vi "SwerveMain.vi"   [LabVIEW 2017]
uses:
  <vilib>/Rock Robotics/Network Tables/NT Read Boolean.vi
  SwerveGlobals.vi
types:
  T1 = typedef "WPI_MotorControlDeviceRef.ctl" = cluster{"DeviceStatus":errorcluster, "Type":T2, "PWM":cluster{"PWM Channel":T3, "DeadBand":T4}, "CAN":cluster{"Device Number":u8, "SetOutput VI Ref":variant, "GetOutput VI Ref":variant, "Enable VI Ref":variant, "Disable VI Ref":variant, "Data":variant}, "Invert":bool, "DIO PWM":cluster{"PWM \"Enable\" Channel":T3, "DIOChannel":T5, "PWM Rate":dbl}}
  T2 = typedef "WPI_MotorControlType.ctl" = enum16{"PWM", "CAN", "DIO PWM"}
  T3 = typedef "FPGA_DIOPWMChannel.ctl" = enum8{"PWM 0", "PWM 1", "PWM 2", "PWM 3", "PWM 4", "PWM 5", "PWM 6", "PWM 7", "PWM 8", "PWM 9", "PWM MXP 0", "PWM MXP 1", "PWM MXP 2", "PWM MXP 3", "PWM MXP 4", "PWM MXP 5", "PWM MXP 6", "PWM MXP 7", "PWM MXP 8", "PWM MXP 9", "Invalid"}
  T4 = typedef "WPI_PWMDeadband.ctl" = cluster{"Name":string, "maxPositivePwm":i32, "minPositivePwm":i32, "centerPwm":i32, "maxNegativePwm":i32, "minNegativePwm":i32, "angularRange":u16}
  T5 = typedef "FPGA_DIOChannel.ctl" = enum8{"DIO 0", "DIO 1", "DIO 2", "DIO 3", "DIO 4", "DIO 5", "DIO 6", "DIO 7", "DIO 8", "DIO 9", "DIO MXP 0", "DIO MXP 1", "DIO MXP 2", "DIO MXP 3", "DIO MXP 4", "DIO MXP 5", "DIO MXP 6", "DIO MXP 7", "DIO MXP 8", "DIO MXP 9", "DIO MXP 10", "DIO MXP 11", "DIO MXP 12", "DIO MXP 13", "DIO MXP 14", "DIO MXP 15", "SPI Port CS1", "SPI Port CS2", "SPI Port CS3", "SPI Port MISO", "SPI Port MOSI", "Invalid"}
  T6 = typedef "WPI_AnalogChannelDevRef.ctl" = cluster{"DevStatus":errorcluster, "Analog Channel":T7}
  T7 = typedef "FPGA_AIChannel.ctl" = enum8{"AI 0", "AI 1", "AI 2", "AI 3", "AI MXP 0", "AI MXP 1", "AI MXP 2", "AI MXP 3", "Invalid"}
  T8 = cluster{"MotorControlDevRef":T1, "MotorControlDevRef":T1, "MotorControlDevRef":T1, "MotorControlDevRef":T1}
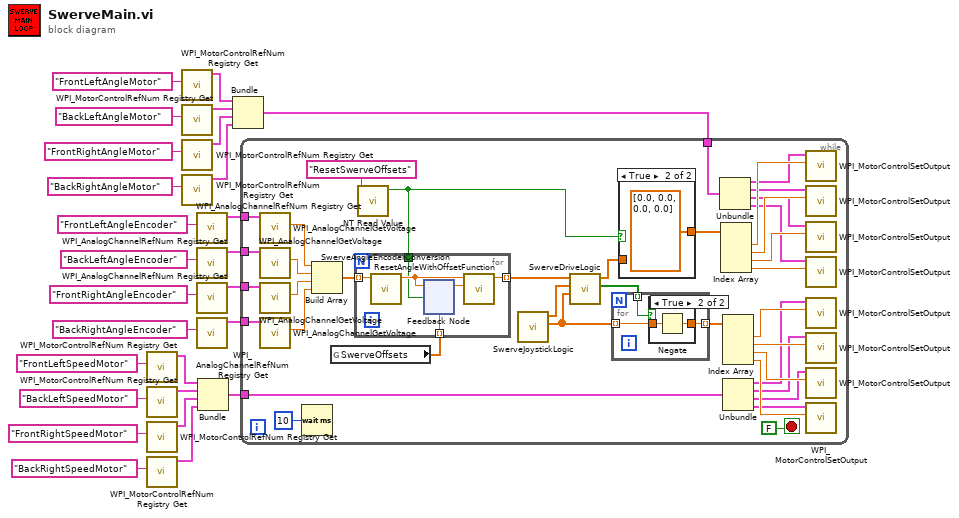
[diagram p0: block diagram]
diagram:
  n1 = call <vilib>:"WPI_MotorControlRefNum Registry Get.vi"("refnum name"="FrontLeftSpeedMotor") -> ("MotorControlDevRef"=w4:T1)  [unwired: 9 in, 1 out]
  n2 = call <vilib>:"WPI_MotorControlRefNum Registry Get.vi"("refnum name"="BackLeftSpeedMotor") -> ("MotorControlDevRef"=w12:T1)  [unwired: 9 in, 1 out]
  n3 = call <vilib>:"WPI_MotorControlRefNum Registry Get.vi"("refnum name"="FrontRightSpeedMotor") -> ("MotorControlDevRef"=w13:T1)  [unwired: 9 in, 1 out]
  n4 = call <vilib>:"WPI_MotorControlRefNum Registry Get.vi"("refnum name"="BackRightSpeedMotor") -> ("MotorControlDevRef"=w14:T1)  [unwired: 9 in, 1 out]
  n5 = call <vilib>:"WPI_MotorControlRefNum Registry Get.vi"("refnum name"="FrontLeftAngleMotor") -> ("MotorControlDevRef"=w1:T1)  [unwired: 9 in, 1 out]
  n6 = call <vilib>:"WPI_MotorControlRefNum Registry Get.vi"("refnum name"="BackLeftAngleMotor") -> ("MotorControlDevRef"=w5:T1)  [unwired: 9 in, 1 out]
  n7 = call <vilib>:"WPI_MotorControlRefNum Registry Get.vi"("refnum name"="FrontRightAngleMotor") -> ("MotorControlDevRef"=w6:T1)  [unwired: 9 in, 1 out]
  n8 = call <vilib>:"WPI_MotorControlRefNum Registry Get.vi"("refnum name"="BackRightAngleMotor") -> ("MotorControlDevRef"=w3:T1)  [unwired: 9 in, 1 out]
  n9 = call <vilib>:"WPI_AnalogChannelRefNum Registry Get.vi"("refnum name"="FrontLeftAngleEncoder") -> ("AIDeviceRef"=w10:T6)  [unwired: 9 in, 1 out]
  n10 = call <vilib>:"WPI_AnalogChannelRefNum Registry Get.vi"("refnum name"="BackLeftAngleEncoder") -> ("AIDeviceRef"=w9:T6)  [unwired: 9 in, 1 out]
  n11 = call <vilib>:"WPI_AnalogChannelRefNum Registry Get.vi"("refnum name"="FrontRightAngleEncoder") -> ("AIDeviceRef"=w8:T6)  [unwired: 9 in, 1 out]
  n12 = call <vilib>:"WPI_AnalogChannelRefNum Registry Get.vi"("refnum name"="BackRightAngleEncoder") -> ("AIDeviceRef"=w7:T6)  [unwired: 9 in, 1 out]
  n13 = Bundle("MotorControlDevRef"=w4, "MotorControlDevRef"=w12, "MotorControlDevRef"=w13, "MotorControlDevRef"=w14) -> (w11:T8)  [unwired: 1 in]
  n14 = Bundle("MotorControlDevRef"=w1, "MotorControlDevRef"=w5, "MotorControlDevRef"=w6, "MotorControlDevRef"=w3) -> (w2:T8)  [unwired: 1 in]
  n15 = while {
    tunnel: w11 -> [w40]
    tunnel: w10 -> [w64]
    tunnel: w9 -> [w63]
    tunnel: w8 -> [w62]
    tunnel: w7 -> [w61]
    tunnel: w2 -> [w38]
    stop <- FALSE stop-if-true
    n16 = call <vilib>:"WPI_AnalogChannelGetVoltage.vi"("AIDeviceRef"=w64) -> ("Voltage"=w60:dbl)  [unwired: 8 in, 2 out]
    n17 = call <vilib>:"WPI_AnalogChannelGetVoltage.vi"("AIDeviceRef"=w63) -> ("Voltage"=w59:dbl)  [unwired: 8 in, 2 out]
    n18 = call <vilib>:"WPI_AnalogChannelGetVoltage.vi"("AIDeviceRef"=w62) -> ("Voltage"=w58:dbl)  [unwired: 8 in, 2 out]
    n19 = call <vilib>:"WPI_AnalogChannelGetVoltage.vi"("AIDeviceRef"=w61) -> ("Voltage"=w57:dbl)  [unwired: 8 in, 2 out]
    n20 = Wait (ms)(milliseconds to wait=u32 10) -> ()  [unwired: 1 out]
    n21 = Build Array(w60, w59, w58, w57) -> (w37:dbl[])
    n22 = global read "SwerveGlobals.vi" "SwerveOffsets"() -> (w35:dbl[])
    n23 = call-poly <vilib>:"NT Read Value.vi"("Name"="ResetSwerveOffsets") -> ("Boolean"=w30:bool)  [unwired: 9 in, 1 out]
    n24 = for {
      tunnel: w37 -> [w73] mode=indexing
      tunnel: w35 -> [w72] mode=indexing
      tunnel: [w69] -> w34 mode=indexing
      tunnel: w30 -> [w68]
      n25 = call "SwerveAngleEncoderConversion.vi"("Voltage"=w73) -> ("Angle"=w71:dbl)  [unwired: 10 in]
      n26 = feedback #1(w72) -> (w70:dbl)
      n27 = feedback-in #1(w71, w68) -> ()
      n28 = call "ResetAngleWithOffsetFunction.vi"("Offset"=w70, "AngleInput"=w71) -> ("AngleOutput"=w69:dbl)  [unwired: 9 in]
    }
    n29 = call "SwerveJoystickLogic.vi"() -> ("Speeds"=w29:dbl[], "Angles"=w33:dbl[])  [unwired: 9 in]
    n30 = call "SwerveDriveLogic.vi"("Speeds"=w29, "AngleSetpoints"=w33, "AngleEncoders"=w34) -> ("AngleMotorsReversed"=w36:bool[], "AngleMotorOutputs"=w32:dbl[])  [unwired: 7 in]
    n31 = for {
      tunnel: w29 -> [w75] mode=indexing
      tunnel: [w76] -> w48 mode=indexing
      tunnel: w36 -> [w74] mode=indexing
      n32 = case shown="True" w74 {
        tunnel: w75 -> [w77 w79]
        tunnel: [w77 w78] -> w76
        frame False {
        }
        frame True {
          n33 = Negate(x=w79) -> (-x=w78:dbl)
        }
      }
    }
    n34 = case shown="True" w30 {
      tunnel: w32 -> [w66 _]
      tunnel: [w66 dbl[] [0.0, 0.0, 0.0, 0.0]] -> w31
      frame False {
      }
      frame True {
      }
    }
    n35 = Unbundle(w38) -> ("MotorControlDevRef"=w51:T1, "MotorControlDevRef"=w50:T1, "MotorControlDevRef"=w49:T1, "MotorControlDevRef"=w41:T1)
    n36 = Index Array(array=w31) -> (element #1=w55:dbl, element #2=w54:dbl, element #3=w53:dbl, element #4=w52:dbl)  [unwired: 4 in]
    n37 = Index Array(array=w48) -> (element #1=w28:dbl, element #2=w46:dbl, element #3=w45:dbl, element #4=w47:dbl)  [unwired: 4 in]
    n38 = Unbundle(w40) -> ("MotorControlDevRef"=w27:T1, "MotorControlDevRef"=w44:T1, "MotorControlDevRef"=w43:T1, "MotorControlDevRef"=w42:T1)
    n39 = call <vilib>:"WPI_MotorControlSetOutput.vi"("Output"=w55, "MotorControlDevRef"=w51) -> ()  [unwired: 7 in, 3 out]
    n40 = call <vilib>:"WPI_MotorControlSetOutput.vi"("Output"=w54, "MotorControlDevRef"=w50) -> ()  [unwired: 7 in, 3 out]
    n41 = call <vilib>:"WPI_MotorControlSetOutput.vi"("Output"=w53, "MotorControlDevRef"=w49) -> ()  [unwired: 7 in, 3 out]
    n42 = call <vilib>:"WPI_MotorControlSetOutput.vi"("Output"=w52, "MotorControlDevRef"=w41) -> ()  [unwired: 7 in, 3 out]
    n43 = call <vilib>:"WPI_MotorControlSetOutput.vi"("Output"=w28, "MotorControlDevRef"=w27) -> ()  [unwired: 7 in, 3 out]
    n44 = call <vilib>:"WPI_MotorControlSetOutput.vi"("Output"=w46, "MotorControlDevRef"=w44) -> ()  [unwired: 7 in, 3 out]
    n45 = call <vilib>:"WPI_MotorControlSetOutput.vi"("Output"=w45, "MotorControlDevRef"=w43) -> ()  [unwired: 7 in, 3 out]
    n46 = call <vilib>:"WPI_MotorControlSetOutput.vi"("Output"=w47, "MotorControlDevRef"=w42) -> ()  [unwired: 7 in, 3 out]
  }
